vi "Set font color of buttons.vi"(8 "error in (no error)":errorcluster, 9 "index":i32, 10 "Values":T1[](array[typedef]), 11 "Ctrl Ref":refnum<vi>) -> (0 "error out":errorcluster)   [LabVIEW 2011]
uses:
  Measurments Handling/Status Digitalish.ctl
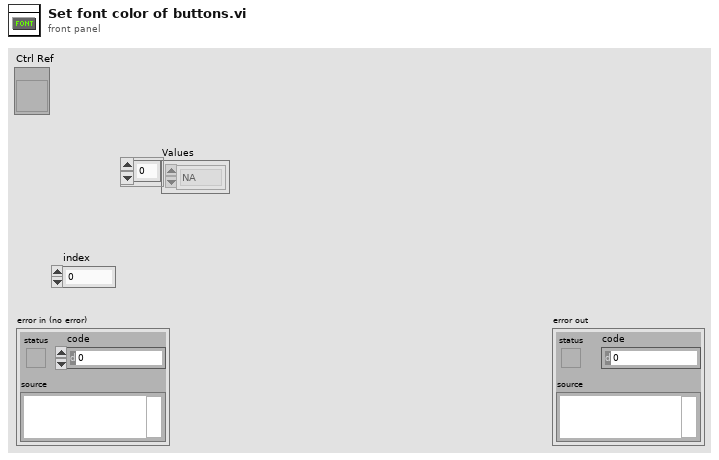
[diagram p1: front panel]
types:
  T1 = typedef "Status Digitalish.ctl" = enum16{"NA", "False", "True"}
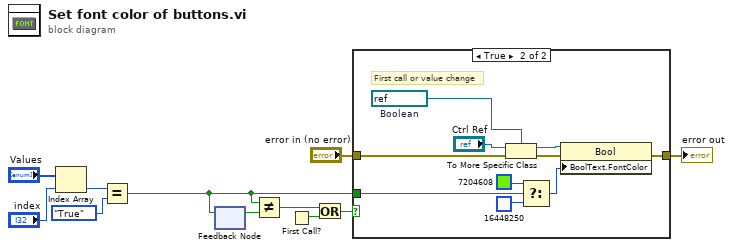
[diagram p0: block diagram]
diagram:
  n1 = Index Array(array="Values", index="index") -> (element=w3:T1)
  n2 = Equal?(x=w3, y=Status_Digitalish."True" ("element")) -> (x = y?=w4:bool)
  n3 = feedback-in #1(w4) -> ()
  n4 = feedback #1() -> (w9:bool)  [unwired: 1 in]
  n5 = Not Equal?(x=w4, y=w9) -> (x != y?=w7:bool)
  n6 = First Call?() -> (First Call?: T/F=w8:bool)
  n7 = Or(x=w7, y=w8) -> (x .or. y?=w6:bool)
  n8 = case shown="True" w6 {
    tunnel: "error in (no error)" -> [w12 w20]
    tunnel: [w12 w16] -> w10
    tunnel: w4 -> [_ w18]
    frame False {
    }
    frame True {
      w22 = refnum<vi> refnum  # Boolean
      # "First call or value change"
      n9 = To More Specific Class(target class=w22, reference="Ctrl Ref", error in=w20) -> (specific class reference=w15:refnum<vi>, error out=w14:errorcluster)
      n10 = Select(t=u32 7204608, s=w18, f=u32 16448250) -> (s? t:f=w13:u32)
      n11 = property on="Property Node" class="Bool"(reference=w15, error in=w14, "BoolText.FontColor"=w13) -> (error out=w16:errorcluster)  [unwired: 1 out]
    }
  }
  "error out" <- w10
